vi "SEScounter.vi"() -> ()   [LabVIEW 2015]
uses:
  <userlib>/caLab/Private/Get_PV-1D.vi
  <userlib>/caLab/Private/Get_PV.vi
  <userlib>/caLab/Private/Put_DBL_PV.vi
  <userlib>/caLab/Private/Put_DBL-1D_PV-1D.vi
panel:
  out "SES:KineticEnergyOrg":dbl=350.0 min=50.0 max=1000.0
  in  "Tab Control":enum32{"Main", "SES:Area", "Stat"}(tab)
  out "Waveform Chart 2":dbl(graph)
  out "Waveform Chart":dynamicdata(graph)
  out "BL132:Io":dbl format="%#_3g"
  out "SES:Area small":i64
  out "SPEAR:State":string
  out "Photon[Hz]":dbl format="%#_3e"
  out "Photon/atom [Hz]":dbl format="%#_3f"
  out "Power[W]":dbl format="%_2g"
  out "SPEC:mono132":dbl format="%_5g"
  out "wavelength/nm":dbl format="%_2g"
  out "SPEC:gap":dbl format="%_2g"
  out "EntSlit":dbl format="%_2g"
  out "ExtSlit":dbl format="%_2g"
  out "SPEC:epu":dbl format="%_2g"
  out "SPEC:sgmensz":dbl format="%_2g"
  out "APX:Theater":dbl format="%_2g"
  out "APX:PiezoX":dbl format="%_2g"
  out "APX:PiezoY":dbl format="%_2g"
  out "APX:PiezoZ":dbl format="%_2g"
  out "SES:BUSY":bool
  out "Fluence[W/cm2]":dbl format="%_2g"
  out "Fluence[uJ/cm2/pulse]":dbl format="%_2g"
  out "SES:Area N":dbl
  out "Theater":dbl
  out "HPC100":dbl
  out "SES:Area":i64
  out "error out":errorcluster
  out "SPEC:ExpNumber_RQ":bool
  out "SPEC:ExpNumber_RV":dbl
  out "SPEC:mono132_RV":dbl
  out "SPEC:OptCH_RV":dbl
  out "SPEC:BUSY":bool
  out "SPEC:OptCH_RQ":bool
  out "SPEC:INC":bool
  out "SPEC:Move_RQ":bool
  out "SES:KineticEnergyValueChage":bool
  out "SES:CalOn_RQ":bool
  out "SES:Run_RQ":bool
  out "SES:Stop_RQ":bool
  out "SES:CalOff_RQ":bool
  out "SPEAR:STATE_OK":bool
  in  "stop":bool
  in  "SES:KineticEnergy":dbl=350.0 min=50.0 max=1000.0
  # "SES-100 slit 0.8mm"
  # "SES partial count-> /Dev/Ctr0 -> /Dev5/PFI14 -> Dev5/ctr1"
  # "Use NI MAX to assing PFI14 as ctr0 output"
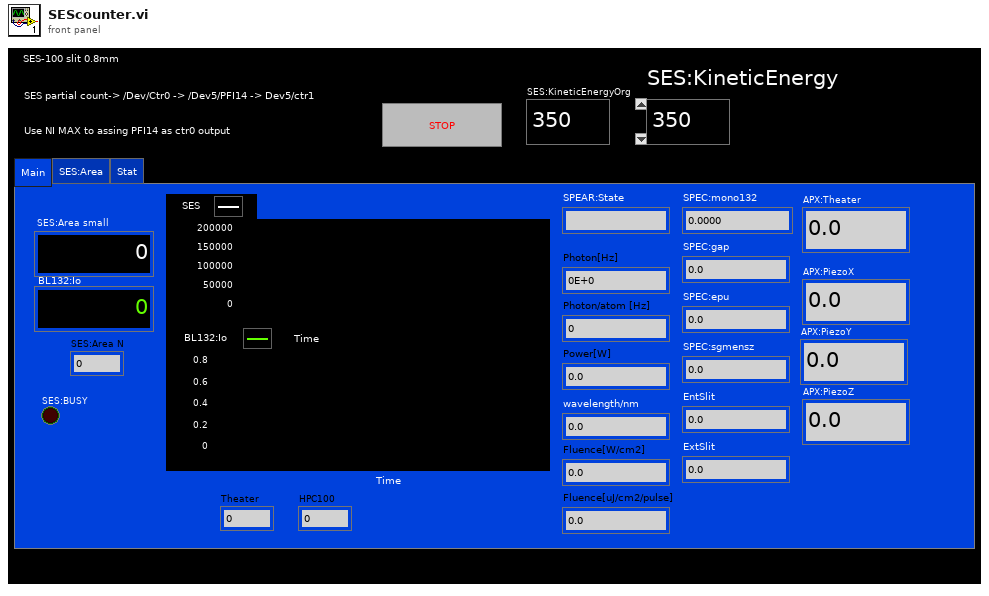
[diagram p1: front panel]
types:
  T1 = enum16{"NO", "SHIFT", "CTRL", "ALT", "SHIFT + CTRL", "SHIFT + ALT", "CTRL + ALT", "SHIFT + CTRL + ALT"}
  T2 = enum16{"Mouse Left", "Mouse Right", "Break", "Mouse Middle", "Backspace", "Tabulator", "FormFeed", "Return", "Shift", "Control", "Alternate", "Pause", "CapsLock", "Escape", "Space", "Page Up", "Page Down", "End", "Home", "Left", "Up", "Right", "Down", "Select", "Print", "Execute", "Snapshot", "Insert", "Delete", "Help", "0", "1", "2", "3", "4", "5", "6", "7", "8", "9", "A", "B", "C", "D", "E", "F", "G", "H", "I", "J", "K", "L", "M", "N", "O", "P", "Q", "R", "S", "T", "U", "V", "W", "X", "Y", "Z", "Win Left", "Win Right", "Context Menu", "Num 0", "Num 1", "Num 2", "Num 3", "Num 4", "Num 5", "Num 6", "Num 7", "Num 8", "Num 9", "Multiply", "Add", "Separator", "Subtract", "Decimal", "Divide", "F1", "F2", "F3", "F4", "F5", "F6", "F7", "F8", "F9", "F10", "F11", "F12", "F13", "F14", "F15", "F16", "F17", "F18", "F19", "F20", "F21", "F22", "F23", "F24", "NumLock", "Scroll", "Shift Left", "Shift Right", "Control Left", "Control Right", "Alternate Left", "Alternate Right", "Attn", "CrSel", "ExSel", "ErEOF", "Play", "Zoom", "Noname", "PA1", "OEM Clear", "Germany <", "Germany ^", "Germany ß", "Germany ´", "Germany ü", "Germany +", "Germany ö", "Germany ä", "Germany #", "Germany ,", "Germany .", "Germany -"}
  T3 = typedef "WindowHandle" = refnum<k1>
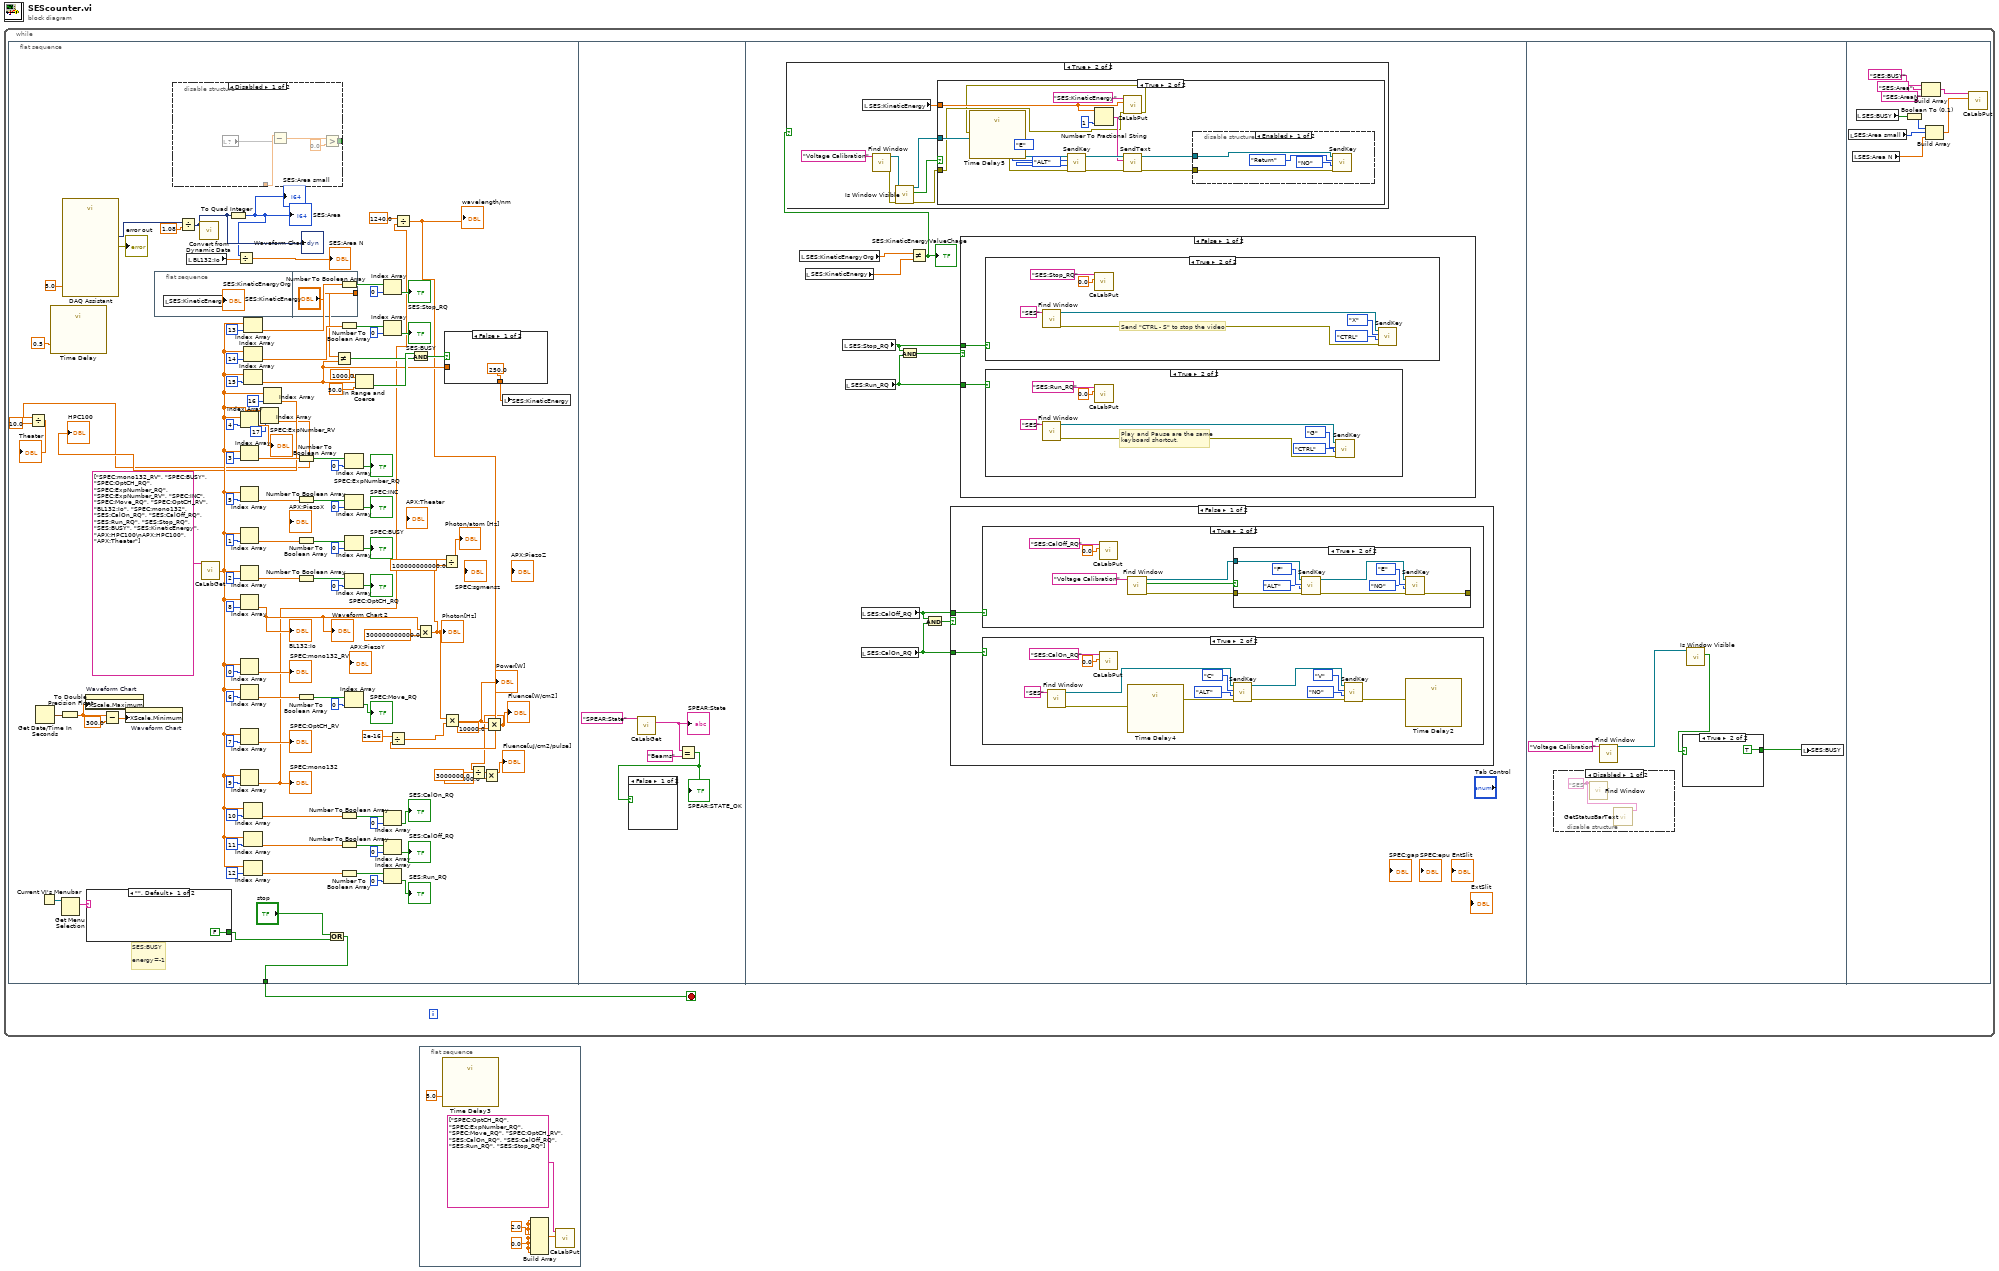
[diagram p0: block diagram]
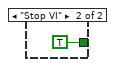
[diagram p4: hidden frame]
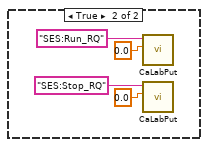
[diagram p11: hidden frame]
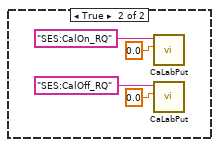
[diagram p15: hidden frame]
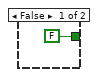
[diagram p17: hidden frame]
diagram:
  n1 = while {
    stop <- w1 stop-if-true
    n2 = flat-sequence {
      tunnel: [w32] -> w1
      frame #0 {
        # "SES:BUSY\n\nenergy=-1"
        n3 = Get Date/Time In Seconds() -> (seconds since 1Jan1904=w109:timestamp)
        n4 = Current VI's Menubar() -> (w111:refnum<k9>)
        n5 = call "Time Delay"("Delay Time (s)"=0.5) -> ()  [unwired: 10 in, 1 out]
        n6 = To Double Precision Float(number=w109) -> (double precision float=w107:dbl)
        n7 = Get Menu Selection(0:w111) -> (6:w110:string)  [unwired: 3 in, 4 out]
        n8 = call "DAQ Assistant"("timeout (s)"=5.0) -> ("data"=w39:dynamicdata, "error out"=→"error out":errorcluster)  [unwired: 16 in, 1 out]
        n9 = property on="Waveform Chart" class="WFChart (strict)"("XScale.Maximum"=w107) -> ()  [unwired: 2 in, 2 out]
        n10 = case shown="\"\", Default" w110 {
          tunnel: [FALSE TRUE] -> w34
          frame "", Default {
          }
          frame "Stop VI" {
          }
        }
        n11 = Subtract(x=w107, y=300.0) -> (x-y=w108:dbl)
        n12 = property on="Waveform Chart" class="WFChart (strict)"("XScale.Minimum"=w108) -> ()  [unwired: 2 in, 2 out]
        n13 = flat-sequence {
          tunnel: ["SES:KineticEnergy"] -> w29
          frame #0 {
            n14 = local read "SES:KineticEnergy"() -> (→"SES:KineticEnergyOrg":dbl)
          }
          frame #1 {
          }
        }
        n15 = disable-structure shown="Disabled" {
          disable-tunnel: _ -> [w116 _]
          disable-tunnel: [w112 _] -> _
          frame Disabled {
            n16 = local read item#-1() -> (w115)
            n17 = Subtract(x=w116, y=w115) -> (x-y=w114:dbl)
            n18 = Greater?(x=w114, y=0.0) -> (0:w112:bool)
          }
          frame Enabled {
          }
        }
        n19 = Divide(x=w39, y=1.08) -> (x/y=w37:dynamicdata)
        "Waveform Chart" <- w37
        n20 = local read "BL132:Io"() -> (w10:dbl)
        n21 = call "Convert from Dynamic Data"("Dynamic Data Type"=w37) -> ()  [unwired: 3 in, 1 out]
        n22 = call-poly <userlib>:"CaLabGet.vi"("PV Names"=string[] ["SPEC:mono132_RV", "SPEC:BUSY", "SPEC:OptCH_RQ", "SPEC:ExpNumber_RQ", "SPEC:ExpNumber_RV", "SPEC:INC", "SPEC:Move_RQ", "SPEC:OptCH_RV", "BL132:Io", "SPEC:mono132", "SES:CalOn_RQ", "SES:CalOff_RQ", "SES:Run_RQ", "SES:Stop_RQ", "SES:BUSY", "SES:KineticEnergy", "APX:HPC100\nAPX:HPC100", "APX:Theater"]) -> ("1rst Value (number)"=w6:dbl[])  [unwired: 8 in, 6 out]
        n23 = To Quad Integer(1:w37) -> (0:w11:i64)
        "SES:Area" <- w11
        "SES:Area small" <- w11
        n24 = Divide(x=w11, y=w10) -> (x/y=→"SES:Area N":dbl)
        n25 = Index Array(array=w6, index=4 ("index (col)")) -> (element=→"SPEC:ExpNumber_RV":dbl)
        n26 = Index Array(array=w6, index=3 ("index (col)")) -> (element=w93:dbl)
        n27 = Index Array(array=w6, index=5 ("index (col)")) -> (element=w90:dbl)
        n28 = Index Array(array=w6, index=1 ("disabled index (col)")) -> (element=w105:dbl)
        n29 = Index Array(array=w6, index=2 ("index (col)")) -> (element=w97:dbl)
        n30 = Index Array(array=w6, index=8) -> (element=w31:dbl)
        "BL132:Io" <- w31
        "Waveform Chart 2" <- w31
        n31 = Index Array(array=w6, index=0 ("disabled index (col)")) -> (element=→"SPEC:mono132_RV":dbl)
        n32 = Index Array(array=w6, index=6 ("index (col)")) -> (element=w83:dbl)
        n33 = Index Array(array=w6, index=7 ("disabled index (col)")) -> (element=→"SPEC:OptCH_RV":dbl)
        n34 = Index Array(array=w6, index=9 ("disabled index (col)")) -> (element=w23:dbl)
        "SPEC:mono132" <- w23
        n35 = Index Array(array=w6, index=13 ("disabled index (col)")) -> (element=w48:dbl)
        n36 = Index Array(array=w6, index=14 ("disabled index (col)")) -> (element=w47:dbl)
        n37 = Index Array(array=w6, index=15 ("disabled index (col)")) -> (element=w41:dbl)
        n38 = Index Array(array=w6, index=10 ("disabled index (col)")) -> (element=w51:dbl)
        n39 = Index Array(array=w6, index=11 ("disabled index (col)")) -> (element=w50:dbl)
        n40 = Index Array(array=w6, index=12 ("disabled index (col)")) -> (element=w49:dbl)
        n41 = Index Array(array=w6, index=17) -> (element=w3:dbl)
        n42 = Divide(x=w3, y=10.0) -> (x/y=→"Theater":dbl)
        n43 = Index Array(array=w6, index=16) -> (element=→"HPC100":dbl)
        n44 = Number To Boolean Array(number=w93) -> (Boolean array=w96:bool[])
        n45 = Number To Boolean Array(number=w90) -> (Boolean array=w92:bool[])
        n46 = Number To Boolean Array(number=w105) -> (Boolean array=w104:bool[])
        n47 = Number To Boolean Array(number=w97) -> (Boolean array=w100:bool[])
        n48 = Number To Boolean Array(number=w83) -> (Boolean array=w86:bool[])
        n49 = Or(x="stop", y=w34) -> (x .or. y?=w32:bool)
        n50 = Not Equal?(x=w29, y=w41) -> (x != y?=w42:bool)
        n51 = Number To Boolean Array(number=w48) -> (Boolean array=w65:bool[])
        n52 = Number To Boolean Array(number=w47) -> (Boolean array=w63:bool[])
        n53 = Number To Boolean Array(number=w51) -> (Boolean array=w71:bool[])
        n54 = Number To Boolean Array(number=w50) -> (Boolean array=w69:bool[])
        n55 = Number To Boolean Array(number=w49) -> (Boolean array=w67:bool[])
        n56 = Index Array(array=w96, index=0) -> (element=→"SPEC:ExpNumber_RQ":bool)
        n57 = Index Array(array=w92, index=0) -> (element=→"SPEC:INC":bool)
        n58 = Index Array(array=w104, index=0) -> (element=→"SPEC:BUSY":bool)
        n59 = Index Array(array=w100, index=0) -> (element=→"SPEC:OptCH_RQ":bool)
        n60 = Index Array(array=w86, index=0) -> (element=→"SPEC:Move_RQ":bool)
        n61 = In Range and Coerce(upper limit=1000.0, x=w41, lower limit=50.0) -> (In Range?=w43:bool)  [unwired: 1 out]
        n62 = Index Array(array=w65, index=0) -> (element=→"SES:Stop_RQ":bool)
        n63 = Index Array(array=w63, index=0) -> (element=→"SES:BUSY":bool)
        n64 = Index Array(array=w71, index=0) -> (element=→"SES:CalOn_RQ":bool)
        n65 = Index Array(array=w69, index=0) -> (element=→"SES:CalOff_RQ":bool)
        n66 = Index Array(array=w67, index=0) -> (element=→"SES:Run_RQ":bool)
        n67 = Divide(x=1240.0, y=w23) -> (x/y=w24:dbl)
        "wavelength/nm" <- w24
        n68 = Divide(x=2e-16, y=w24) -> (x/y=w26:dbl)
        n69 = And(x=w43, y=w42) -> (x .and. y?=w40:bool)
        n70 = Multiply(x=w31, y=300000000000.0) -> (x*y=w22:dbl)
        "Photon[Hz]" <- w22
        n71 = Divide(x=w22, y=100000000000.0) -> (x/y=→"Photon/atom [Hz]":dbl)
        n72 = Multiply(x=w22, y=w26) -> (x*y=w19:dbl)
        "Power[W]" <- w19
        n73 = case shown="False" w40 {
          tunnel: w41 -> [_ w120]
          tunnel: [250.0 w120] -> w12
          frame False {
          }
          frame True {
          }
        }
        n74 = Multiply(x=w19, y=10000.0) -> (x*y=w17:dbl)
        "Fluence[W/cm2]" <- w17
        n75 = Divide(x=w17, y=3000000.0) -> (x/y=w16:dbl)
        n76 = Multiply(x=w16, y=1000000.0) -> (x*y=→"Fluence[uJ/cm2/pulse]":dbl)
        n77 = local write "SES:KineticEnergy"(w12) -> ()
      }
      frame #1 {
        n78 = call-poly <userlib>:"CaLabGet.vi"("PV Name"="SPEAR:State") -> ("1rst Value (string)"=w124:string)  [unwired: 8 in, 6 out]
        "SPEAR:State" <- w124
        n79 = Equal?(x=w124, y="Beams") -> (x = y?=w126:bool)
        "SPEAR:STATE_OK" <- w126
        n80 = case shown="False" w126 {
          frame False {
          }
          frame True {
          }
        }
      }
      frame #2 {
        n81 = local read "SES:KineticEnergyOrg"() -> (w129:dbl)
        n82 = local read "SES:KineticEnergy"() -> (w128:dbl)
        n83 = local read "SES:Stop_RQ"() -> (w131:bool)
        n84 = local read "SES:Run_RQ"() -> (w130:bool)
        n85 = local read "SES:CalOff_RQ"() -> (w133:bool)
        n86 = local read "SES:CalOn_RQ"() -> (w134:bool)
        n87 = And(x=w131, y=w130) -> (x .and. y?=w132:bool)
        n88 = Not Equal?(x=w129, y=w128) -> (x != y?=w127:bool)
        "SES:KineticEnergyValueChage" <- w127
        n89 = case shown="True" w127 {
          frame False {
          }
          frame True {
            n90 = local read "SES:KineticEnergy"() -> (w141:dbl)
            n91 = call "Find Window.vi"("WindowName"="Voltage Calibration") -> ("error out"=w137:errorcluster, "WindowHandle"=w140:T3)  [unwired: 8 in, 1 out]
            n92 = call "Is Window Visible.vi"("error in (no error)"=w137, "WindowHandleIn"=w140) -> ("error out"=w136:errorcluster, "WindowVisible"=w138:bool, "WindowHandle"=w139:T3)  [unwired: 7 in]
            n93 = case shown="True" w138 {
              tunnel: w139 -> [_ w156]
              tunnel: w136 -> [_ w144]
              tunnel: w141 -> [_ w146]
              frame False {
              }
              frame True {
                n94 = Number To Fractional String(number=w146, precision (6)=i16 1) -> (F-format string=w148:string)  [unwired: 2 in]
                n95 = call-poly <userlib>:"CaLabPut.vi"("Error in (no error)"=w144, "Value"=w146, "PV Name"="SES:KineticEnergy") -> ("Error out"=w143:errorcluster)  [unwired: 5 in, 3 out]
                n96 = call "Time Delay5"("error in (no error)"=w143) -> ("error out"=w145:errorcluster)  [unwired: 10 in]
                n97 = call "SendKey.vi"("error in (no error)"=w145, "ShiftState"=T1."ALT", "Virtual Key"=T2."E", "WindowHandle"=w156) -> ("error out"=w152:errorcluster, "Previous WindowHandle"=w153:T3)  [unwired: 2 in]
                n98 = call "SendText.vi"("error in (no error)"=w152, "Text"=w148, "WindowHandle"=w153) -> ("error out"=w150:errorcluster, "Previous WindowHandle"=w151:T3)  [unwired: 3 in]
                n99 = disable-structure shown="Enabled" {
                  disable-tunnel: w151 -> [w160 _]
                  disable-tunnel: w150 -> [w157 _]
                  frame Enabled {
                    n100 = call "SendKey.vi"("error in (no error)"=w157, "ShiftState"=T1."NO", "Virtual Key"=T2."Return", "WindowHandle"=w160) -> ()  [unwired: 2 in, 2 out]
                  }
                  frame Disabled {
                  }
                }
              }
            }
          }
        }
        n101 = And(x=w133, y=w134) -> (x .and. y?=w135:bool)
        n102 = case shown="False" w135 {
          tunnel: w134 -> [w182 _]
          tunnel: w133 -> [w181 _]
          frame False {
            n103 = case shown="True" w181 {
              frame False {
              }
              frame True {
                n104 = call-poly <userlib>:"CaLabPut.vi"("Value"=0.0, "PV Name"="SES:CalOff_RQ") -> ()  [unwired: 6 in, 4 out]
                n105 = call "Find Window.vi"("WindowName"="Voltage Calibration") -> ("error out"=w185:errorcluster, "WindowFound"=w186:bool, "WindowHandle"=w184:T3)  [unwired: 8 in]
                n106 = case shown="True" w186 {
                  tunnel: w184 -> [_ w198]
                  tunnel: w185 -> [w189 w195]
                  tunnel: [w189 w190] -> _
                  frame False {
                  }
                  frame True {
                    n107 = call "SendKey.vi"("error in (no error)"=w195, "ShiftState"=T1."ALT", "Virtual Key"=T2."F", "WindowHandle"=w198) -> ("error out"=w191:errorcluster, "Previous WindowHandle"=w192:T3)  [unwired: 2 in]
                    n108 = call "SendKey.vi"("error in (no error)"=w191, "ShiftState"=T1."NO", "Virtual Key"=T2."E", "WindowHandle"=w192) -> ("error out"=w190:errorcluster)  [unwired: 2 in, 1 out]
                  }
                }
              }
            }
            n109 = case shown="True" w182 {
              frame False {
              }
              frame True {
                n110 = call "Find Window.vi"("WindowName"="SES") -> ("error out"=w200:errorcluster, "WindowHandle"=w201:T3)  [unwired: 8 in, 1 out]
                n111 = call-poly <userlib>:"CaLabPut.vi"("Value"=0.0, "PV Name"="SES:CalOn_RQ") -> ()  [unwired: 6 in, 4 out]
                n112 = call "Time Delay4"("error in (no error)"=w200) -> ("error out"=w199:errorcluster)  [unwired: 10 in]
                n113 = call "SendKey.vi"("error in (no error)"=w199, "ShiftState"=T1."ALT", "Virtual Key"=T2."C", "WindowHandle"=w201) -> ("error out"=w206:errorcluster, "Previous WindowHandle"=w207:T3)  [unwired: 2 in]
                n114 = call "SendKey.vi"("error in (no error)"=w206, "ShiftState"=T1."NO", "Virtual Key"=T2."V", "WindowHandle"=w207) -> ("error out"=w209:errorcluster)  [unwired: 2 in, 1 out]
                n115 = call "Time Delay2"("error in (no error)"=w209) -> ()  [unwired: 10 in, 1 out]
              }
            }
          }
          frame True {
            n116 = call-poly <userlib>:"CaLabPut.vi"("Value"=0.0, "PV Name"="SES:CalOn_RQ") -> ()  [unwired: 6 in, 4 out]
            n117 = call-poly <userlib>:"CaLabPut.vi"("Value"=0.0, "PV Name"="SES:CalOff_RQ") -> ()  [unwired: 6 in, 4 out]
          }
        }
        n118 = case shown="False" w132 {
          tunnel: w130 -> [w162 _]
          tunnel: w131 -> [w161 _]
          frame False {
            n119 = case shown="True" w161 {
              frame False {
              }
              frame True {
                # "Send \"CTRL - S\" to stop the video"
                n120 = call "Find Window.vi"("WindowName"="SES") -> ("error out"=w172:errorcluster, "WindowHandle"=w173:T3)  [unwired: 8 in, 1 out]
                n121 = call-poly <userlib>:"CaLabPut.vi"("Value"=0.0, "PV Name"="SES:Stop_RQ") -> ()  [unwired: 6 in, 4 out]
                n122 = call "SendKey.vi"("error in (no error)"=w172, "ShiftState"=T1."CTRL", "Virtual Key"=T2."X", "WindowHandle"=w173) -> ()  [unwired: 2 in, 2 out]
              }
            }
            n123 = case shown="True" w162 {
              frame False {
              }
              frame True {
                # "Play and Pause are the same\nkeyboard shortcut."
                n124 = call "Find Window.vi"("WindowName"="SES") -> ("error out"=w165:errorcluster, "WindowHandle"=w166:T3)  [unwired: 8 in, 1 out]
                n125 = call-poly <userlib>:"CaLabPut.vi"("Value"=0.0, "PV Name"="SES:Run_RQ") -> ()  [unwired: 6 in, 4 out]
                n126 = call "SendKey.vi"("error in (no error)"=w165, "ShiftState"=T1."CTRL", "Virtual Key"=T2."G", "WindowHandle"=w166) -> ()  [unwired: 2 in, 2 out]
              }
            }
          }
          frame True {
            n127 = call-poly <userlib>:"CaLabPut.vi"("Value"=0.0, "PV Name"="SES:Run_RQ") -> ()  [unwired: 6 in, 4 out]
            n128 = call-poly <userlib>:"CaLabPut.vi"("Value"=0.0, "PV Name"="SES:Stop_RQ") -> ()  [unwired: 6 in, 4 out]
          }
        }
      }
      frame #3 {
        n129 = disable-structure shown="Disabled" {
          frame Disabled {
            w220 = "SES" ("WindowName")
            n130 = call "Find Window.vi"("WindowName"=w220) -> ()  [unwired: 8 in, 3 out]
            n131 = call "GetStatusBarText.vi"("WindowName"=w220) -> ()  [unwired: 9 in, 2 out]
          }
          frame Enabled {
          }
        }
        n132 = call "Find Window.vi"("WindowName"="Voltage Calibration") -> ("WindowHandle"=w217:T3)  [unwired: 8 in, 2 out]
        n133 = call "Is Window Visible.vi"("WindowHandleIn"=w217) -> ("WindowVisible"=w216:bool)  [unwired: 8 in, 2 out]
        n134 = case shown="True" w216 {
          tunnel: [FALSE TRUE] -> w219
          frame False {
          }
          frame True {
          }
        }
        n135 = local write "SES:BUSY"(w219) -> ()
      }
      frame #4 {
        n136 = local read "SES:Area small"() -> (w228:i64)
        n137 = local read "SES:Area N"() -> (w223:dbl)
        n138 = local read "SES:BUSY"() -> (w231:bool)
        n139 = Boolean To (0,1)(Boolean=w231) -> (0, 1=w229:i16)
        n140 = Build Array("SES:BUSY" ("PV Name"), "SES:Area" ("PV Name"), "SES:AreaN" ("element")) -> (w226:string[])
        n141 = Build Array(w229, w228, w223) -> (w227:dbl[])
        n142 = call-poly <userlib>:"CaLabPut.vi"("Values"=w227, "PV Names"=w226) -> ()  [unwired: 6 in, 4 out]
      }
    }
  }
  n143 = flat-sequence {
    frame #0 {
      w233 = 0.0
      n144 = call "Time Delay3"("Delay Time (s)"=5.0) -> ()  [unwired: 10 in, 1 out]
      n145 = Build Array(w233, w233, w233, 2.0, w233, w233, w233, w233) -> (w234:dbl[])
      n146 = call-poly <userlib>:"CaLabPut.vi"("Values"=w234, "PV Names"=string[] ["SPEC:OptCH_RQ", "SPEC:ExpNumber_RQ", "SPEC:Move_RQ", "SPEC:OptCH_RV", "SES:CalOn_RQ", "SES:CalOff_RQ", "SES:Run_RQ", "SES:Stop_RQ"]) -> ()  [unwired: 6 in, 4 out]
    }
  }
